vi "HEWH Zero Truckated Array.vi"(6 "Zero End Index":i32, 8 "error in (no error)":errorcluster, 9 "Zero Start Index":i32, 10 "Totalized Flow Index":i32, 11 "Test Data-Start to End DBL":dbl[][](array[numeric])) -> (0 "error out":errorcluster, 3 "Test Data-Start to End DBL Output":dbl[][](array[numeric]))   [LabVIEW 2023]
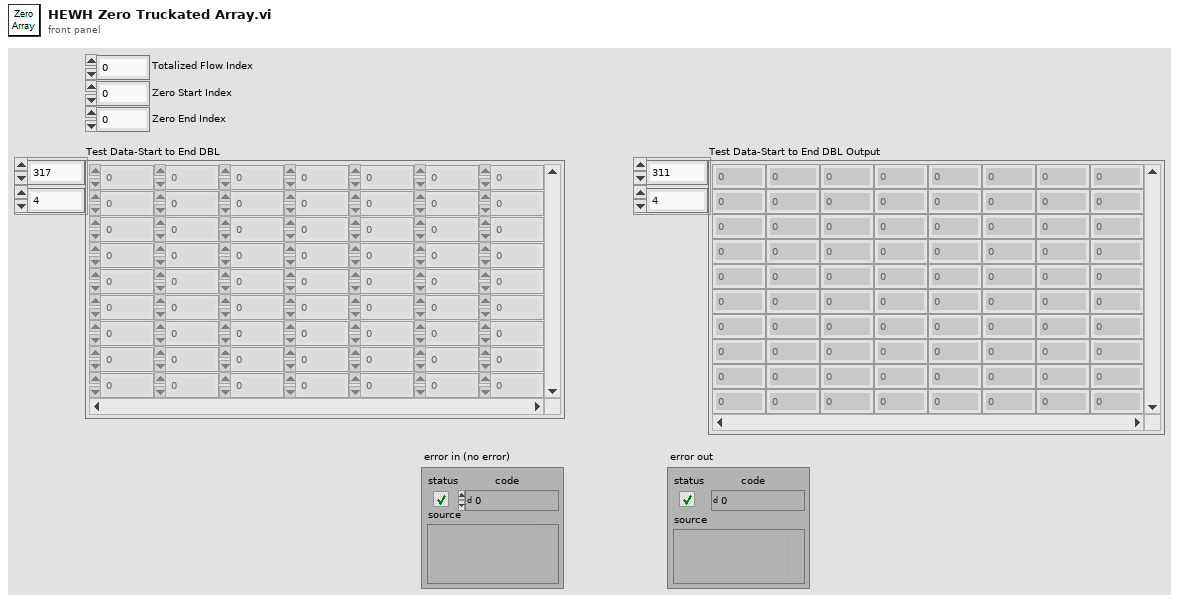
[diagram p1: front panel]
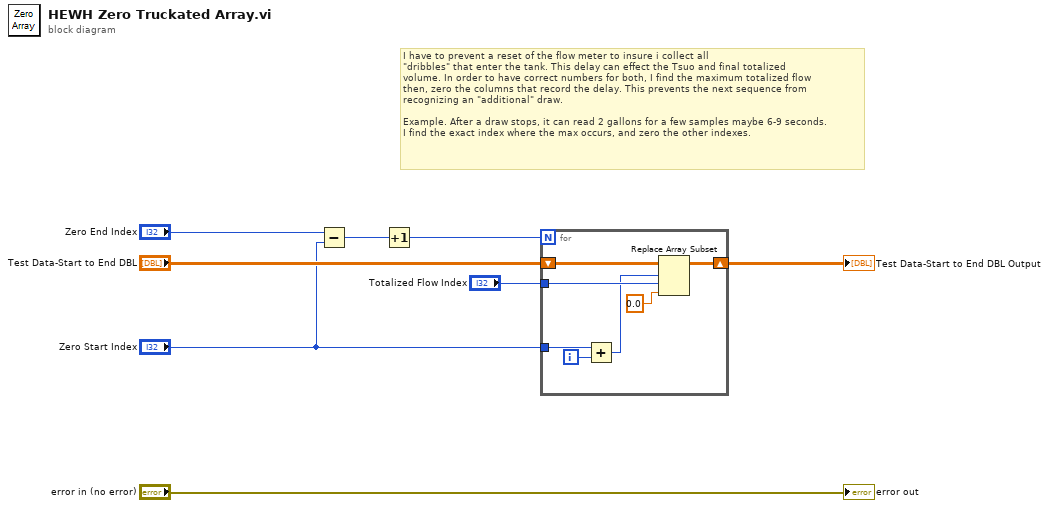
[diagram p0: block diagram]
diagram:
  # "I have to prevent a reset of the flow meter to insure i collect all\n\"dribbles\" that enter the tank. This delay can effect the Tsuo and final totalized \nvolume. In order to have correct numbers for both, I find the maximum totalized flow\nthen, zero the columns that record the delay. This prevents the next sequence from\nrecognizing an \"additional\" draw.\n\nExample. After a draw stops, it can read 2 gallons for a few samples maybe 6-9 seconds.\nI find the exact index where the max occurs, and zero the other indexes."
  n1 = Subtract(x="Zero End Index", y="Zero Start Index") -> (x-y=w2:i32)
  n2 = Increment(x=w2) -> (x+1=w1:i32)
  n3 = for {
    N: w1 -> [_]
    tunnel: "Totalized Flow Index" -> [w15]
    tunnel: "Zero Start Index" -> [w12]
    shift-right: [w9] -> w6
    shift-left: "Test Data-Start to End DBL" -> [w14]
    i -> [w13]
    n4 = Add(x=w12, y=w13) -> (x+y=w11:i32)
    n5 = Replace Array Subset(array=w14, new element=0.0 ("new element/subarray"), index (row)=w11, index (col)=w15) -> (w9:dbl[][])
  }
  "Test Data-Start to End DBL Output" <- w6
  "error out" <- "error in (no error)"
